vi "OSF Read Projects.vi"(6 "Read wikis":bool, 7 "OSF API URL":string="https://api.osf.io/v2/", 8 "error in":errorcluster, 9 "$Path or Item Name":string, 10 "node":string, 11 "client handle":T1) -> (0 "error out":errorcluster, 1 "<JSON>":string[](array[string]) caption="<JSON>Items", 2 "Upload link":string, 3 "client handle out":T1, 4 "body":string, 5 "Wiki ID":string)   [LabVIEW 2020]
uses:
  <vilib>/httpClient/ClientHandle.ctl
  <vilib>/JDP Science/JSONtext/Find Item.vi
  <vilib>/JDP Science/JSONtext/String Subset.vi
  <vilib>/JDP Science/JSONtext/Offset/Find Object Item Locations by Names.vi
  <vilib>/JDP Science/JSONtext/support/Quote and Escape JSON string.vi
  <vilib>/JDP Science/JSONtext/Parsing/Advance past whitespace.vi
  <vilib>/JDP Science/JSONtext/Parsing/Advance past whitespace and comma.vi
  <vilib>/JDP Science/JSONtext/Parsing/Advance past next JSON Value (inlined COPY).vi
  <vilib>/JDP Science/JSONtext/Parsing/Advance past Item Name.vi
  <vilib>/JDP Science/JSONtext/support/quote and escape json string 2.vi
  <vilib>/JDP Science/JSONtext/Parsing/Advance past Line Ending.vi
  <vilib>/JDP Science/JSONtext/Parsing/Advance past String.vi
  <vilib>/JDP Science/JSONtext/Parsing/Advance past Number.vi
  <vilib>/JDP Science/JSONtext/Parsing/Parse Full Path or Item Name.vi
  <vilib>/JDP Science/JSONtext/Next JSON Value.vi
  <vilib>/JDP Science/JSONtext/support/Error Cluster From Code.vi
  <vilib>/JDP Science/JSONtext/Offset/Find Item Locations by Path.vi
  <vilib>/JDP Science/JSONtext/Parsing/Advance past Array.vi
  <vilib>/JDP Science/JSONtext/Parsing/Advance past Object.vi
  <vilib>/JDP Science/JSONtext/Parsing/Parsing Error.vi
  <vilib>/httpClient/LabVIEWHTTPClient.lvlib
  <vilib>/JDP Science/JSONtext/JSONtext.lvlib
panel:
  out "<JSON> 3":string[](array[string]) caption="<JSON>Items"
  out "Item Names":string[](array[string])
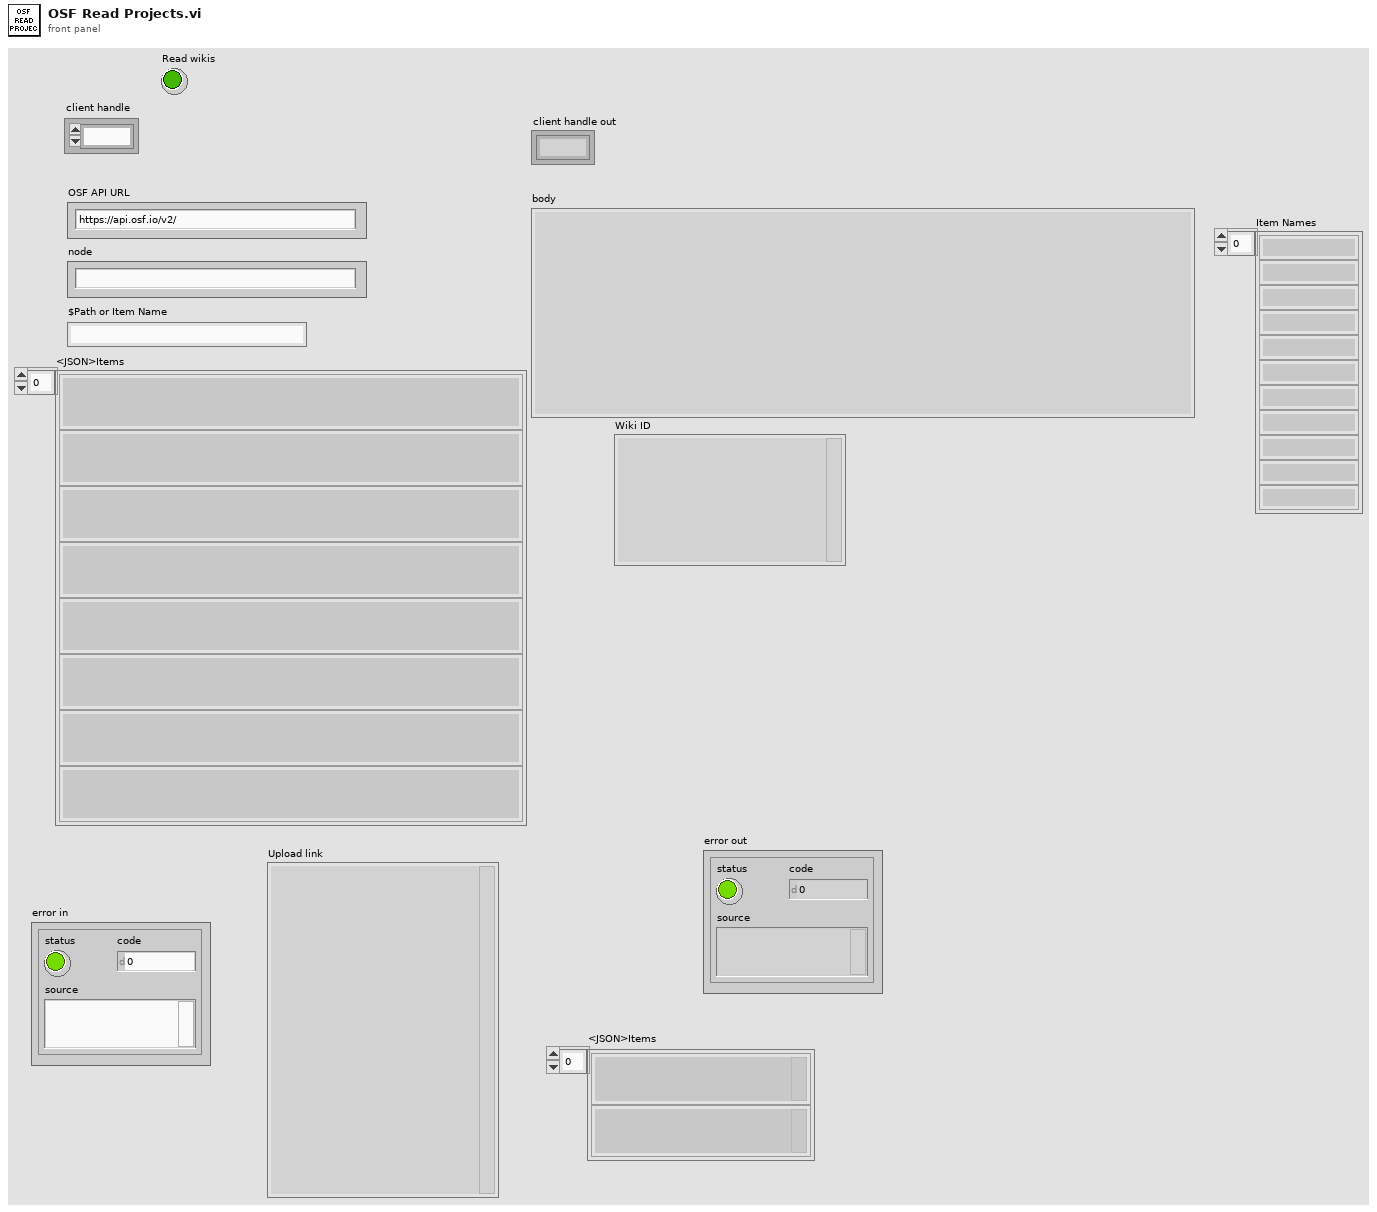
[diagram p1: front panel]
types:
  T1 = typedef "LabVIEWHTTPClient.lvlib/ClientHandle.ctl" = refnum<k1>
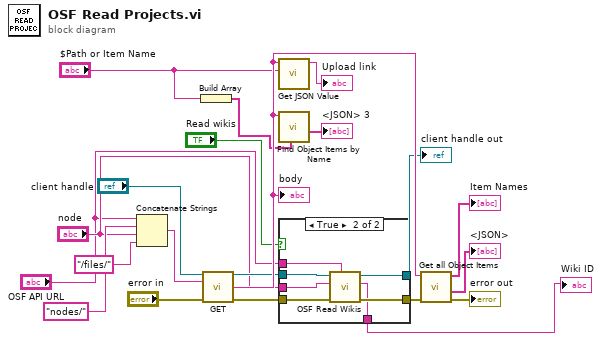
[diagram p0: block diagram]
diagram:
  n1 = Concatenate Strings("OSF API URL", "nodes/", "node", "/files/" ("string")) -> (w20:string)
  n2 = Build Array("$Path or Item Name") -> (w16:string[])
  n3 = call <vilib>:"GET.vi"("client handle"="client handle", "url"=w20, "error in (no error)"="error in") -> ("client handle out"=w9:T1, "body"=w17:string, "error out"=w10:errorcluster)  [unwired: 9 in, 1 out]
  "body" <- w17
  n4 = call "Get JSON Value.vi"("$Path or Item Name"="$Path or Item Name", "JSON in"=w17) -> ("Value"=→"Upload link":string)  [unwired: 6 in, 3 out]
  n5 = call <vilib>:"Find Object Items by Name.vi"("Item Names"=w16, "JSON"=w17) -> ("<JSON>"=→"<JSON> 3":string[])  [unwired: 7 in, 2 out]
  n6 = case shown="True" "Read wikis" {
    tunnel: w10 -> [w22 w30]
    tunnel: [w22 w29] -> w3
    tunnel: w9 -> [w23 w28]
    tunnel: [w23 w27] -> w4
    tunnel: "node" -> [_ w26]
    tunnel: "OSF API URL" -> [_ w25]
    tunnel: [_ w24] -> w1
    frame False {
    }
    frame True {
      n7 = call "OSF Read Wikis.vi"("OSF API URL"=w25, "error in"=w30, "node"=w26, "client handle"=w28) -> ("error out"=w29:errorcluster, "Wiki ID"=w24:string, "client handle out"=w27:T1)  [unwired: 3 in, 2 out]
    }
  }
  "client handle out" <- w4
  "Wiki ID" <- w1
  n8 = call <vilib>:"Get all Object Items.vi"("error in (no error)"=w3, "JSON"=w17) -> ("error out"=→"error out":errorcluster, "<JSON>"=→"<JSON>":string[], "Item Names"=→"Item Names":string[])  [unwired: 6 in, 1 out]
